vi "Actor Core.vi"(8 "error in":errorcluster, 11 "Example Controller":refnum<class "Example Controller.lvclass">) -> (0 "error out":errorcluster, 3 "Actor out":refnum<class "Actor.lvclass">)   [LabVIEW 2023, in "Example GUI View.lvlib" / "Example Controller.lvclass"]
doc: "This is Actor Core.vi, the main message handling loop for Actors. An actor usually just sits in this loop and processes messages as they arrive. Any error returned by the message Do.vi call will stop the loop, with error code 43 as the cannonical signal to stop with no error sent to caller. Descendants may override that in Handle Error.vi."
uses:
  Example Controller.lvclass
  <vilib>/ActorFramework/Actor/Actor.lvclass
  <vilib>/ActorFramework/Message Enqueuer/Message Enqueuer.lvclass
  <vilib>/ActorFramework/Actor/Actor.lvclass/Actor.ctl
  <vilib>/ActorFramework/Message Enqueuer/Message Enqueuer.lvclass/Message Enqueuer.ctl
  Example Controller.lvclass/Example Controller.ctl
  <vilib>/ActorFramework/Message Enqueuer/Init from Existing Queue.vi
  <vilib>/ActorFramework/Message Enqueuer/Enqueue.vi
  <vilib>/ActorFramework/Stop Msg/Stop Msg.lvclass
  <vilib>/Utility/LVClass/Get LV Class Name.vi
  <resource>/AFDebug/Generate Trace for Message.vi
  <vilib>/ActorFramework/Message Priority Queue/Priority Enqueue.vi
  Example Controller/Example Controller/Example Controller.lvclass
  GUI Views/GUI View Messages/Close Front Panel Msg/Close Front Panel Msg.lvclass
  GUI Views/GUI View Messages/Open Front Panel Msg/Open Front Panel Msg.lvclass
  GUI Views/GUI View Messages/Set Front Panel State Msg/Set Front Panel State Msg.lvclass
  <userlib>/_OpenG.lib/error/error.llb/openg_error.lvlib
panel:
  in  "Exit":bool
  in  "Activate?":bool
  in  "Front Panel Window:State":T1(ring)=enum."Standard"
  in  "Set Container FP State":bool
  in  "Close Container FP":bool
  in  "Open Container FP":bool
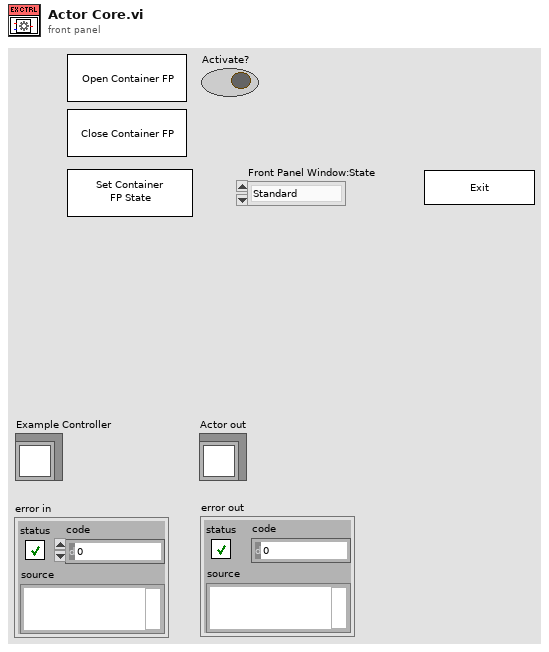
[diagram p1: front panel]
types:
  T1 = enum32{"Invalid", "Standard", "Closed", "Hidden", "Minimized", "Maximized"}
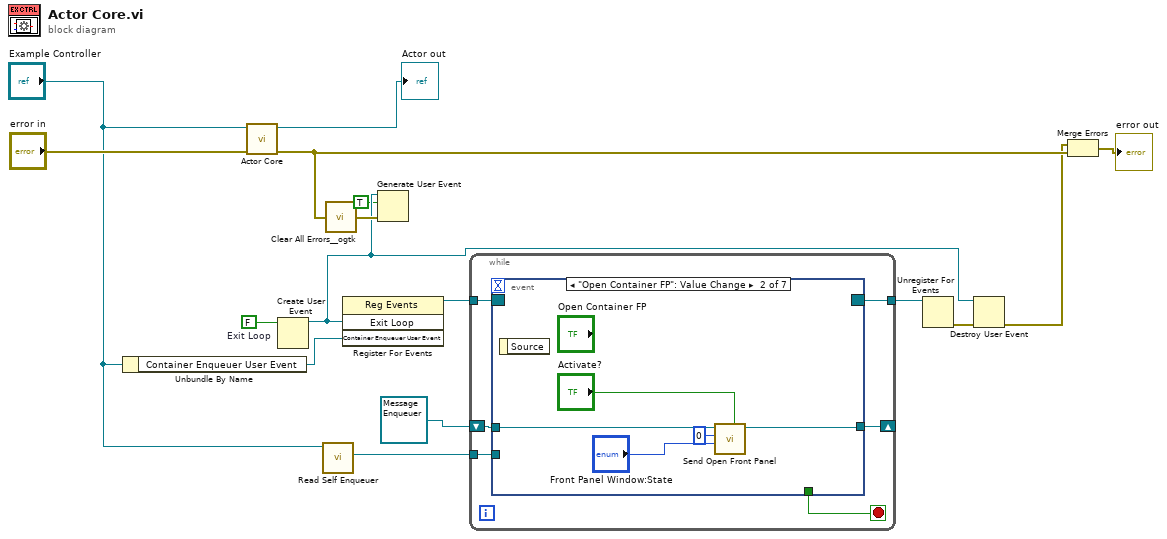
[diagram p0: block diagram]
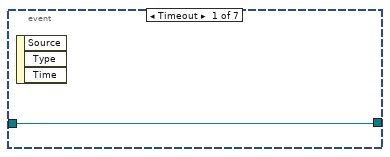
[diagram p2: hidden frame]
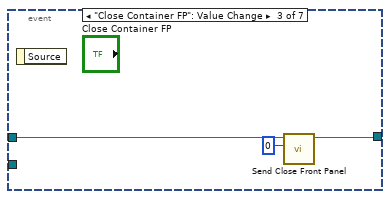
[diagram p3: hidden frame]
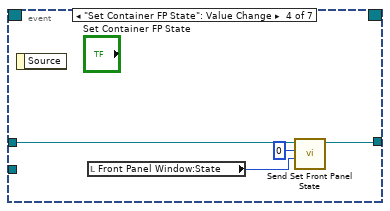
[diagram p4: hidden frame]
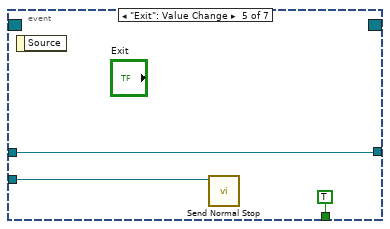
[diagram p5: hidden frame]
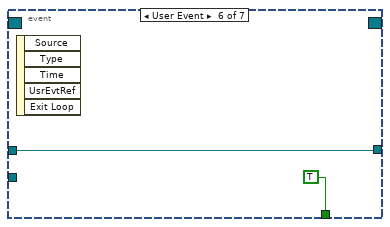
[diagram p6: hidden frame]
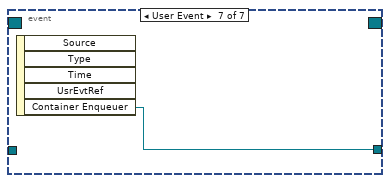
[diagram p7: hidden frame]
diagram:
  w12 = FALSE  # Exit Loop
  n1 = Unbundle By Name("Example Controller") -> ("Container Enqueuer User Event"=w2:refnum<user-event>)
  n2 = call-parent "Actor Core.vi"("error in"="error in", "Example Controller"="Example Controller") -> ("error out"=w8:errorcluster, "Actor out"=→"Actor out":refnum<class "Actor.lvclass">)  [unwired: 8 in]
  n3 = Create User Event(user event datatype=w12) -> (user event=w6:refnum<user-event>)  [unwired: 1 in, 1 out]
  n4 = call <vilib>:"Read Self Enqueuer.vi"("Actor"="Example Controller") -> ("Self Enqueuer"=w13:refnum<class "Message Enqueuer.lvclass">)  [unwired: 10 in]
  n5 = call <userlib>:"Clear All Errors__ogtk.vi"("Error In"=w8) -> ("Error Out"=w7:errorcluster)  [unwired: 3 in]
  n6 = register-events(w6, w2) -> (reference out=w11:refnum<event-registration>)  [unwired: 2 in, 1 out]
  n7 = Generate User Event(user event=w6, event data cluster=TRUE ("event data"), error in=w7) -> ()  [unwired: 1 in, 2 out]
  n8 = while {
    tunnel: w13 -> [w21]
    tunnel: w11 -> [w20]
    tunnel: [w18] -> w10
    shift-right: [w17] -> _
    shift-left: refnum<class "Message Enqueuer.lvclass"> refnum ("Container Enqueuer") -> [w22]
    stop <- w19 stop-if-true
    n9 = event shown="[1] \"Open Container FP\": Value Change" {
      selector: w20 -> [_ _ _ _ _ _ _]
      dyn-events: [_ _ _ _ _ _ _] -> w18
      timeout: _ -> [_ _ _ _ _ _ _]
      tunnel: w22 -> [w23 w28 w30 w35 w36 w39 _]
      tunnel: w21 -> [_ _ _ _ w38 _ _]
      tunnel: [_ _ _ _ TRUE TRUE _] -> w19
      tunnel: [w23 w24 w29 w32 w36 w39 w41] -> w17
      event Timeout {
        n10 = event-data() -> ()  [unwired: 1 in, 3 out]
      }
      event "Open Container FP": Value Change {
        n11 = event-data() -> ()  [unwired: 1 in, 1 out]
        n12 = call "Send Open Front Panel.vi"("Activate?"="Activate?", "Front Panel Window:State"="Front Panel Window:State", "View Hierarchy Level"=0, "Message Enqueuer in"=w28) -> ("Message Enqueuer out"=w24:refnum<class "Message Enqueuer.lvclass">)  [unwired: 6 in, 1 out]
      }
      event "Close Container FP": Value Change {
        n13 = event-data() -> ()  [unwired: 1 in, 1 out]
        n14 = call "Send Close Front Panel.vi"("View Hierarchy Level"=0, "Message Enqueuer in"=w30) -> ("Message Enqueuer out"=w29:refnum<class "Message Enqueuer.lvclass">)  [unwired: 8 in, 1 out]
      }
      event "Set Container FP State": Value Change {
        n15 = event-data() -> ()  [unwired: 1 in, 1 out]
        n16 = local read "Front Panel Window:State"() -> (w33:T1)
        n17 = call "Send Set Front Panel State.vi"("Front Panel Window:State"=w33, "View Hierarchy Level"=0, "Message Enqueuer in"=w35) -> ("Message Enqueuer out"=w32:refnum<class "Message Enqueuer.lvclass">)  [unwired: 7 in, 1 out]
      }
      event "Exit": Value Change {
        n18 = event-data() -> ()  [unwired: 1 in, 1 out]
        n19 = call <vilib>:"Send Normal Stop.vi"("Message Enqueuer"=w38) -> ()  [unwired: 10 in, 1 out]
      }
      event User Event {
        n20 = event-data() -> ()  [unwired: 1 in, 5 out]
      }
      event User Event {
        n21 = event-data() -> ("Container Enqueuer"=w41:refnum<class "Message Enqueuer.lvclass">)  [unwired: 1 in, 4 out]
      }
    }
  }
  n22 = Unregister For Events(event registration refnum=w10) -> (error out=w9:errorcluster)  [unwired: 1 in]
  n23 = Destroy User Event(user event=w6, error in=w9) -> (error out=w3:errorcluster)
  n24 = Merge Errors(w3, w8) -> (→"error out":errorcluster)
